vi "Sort 1D Array.vi"   [LabVIEW 2018]
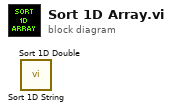
[diagram p0: block diagram]
diagram:
  n1 = call "Sort 1D String.vi"() -> ()  [unwired: 1 in, 1 out]
  n2 = call "Sort 1D Double.vi"() -> ()  [unwired: 1 in, 1 out]
